vi "NeoShutdown.vi"(4 "Error In":errorcluster) -> (0 "ErrorOut":errorcluster)   [LabVIEW 2014]
panel:
  out "Close: status":i32
  out "Status: clear all buffers":i32
  in  "Handle":i32
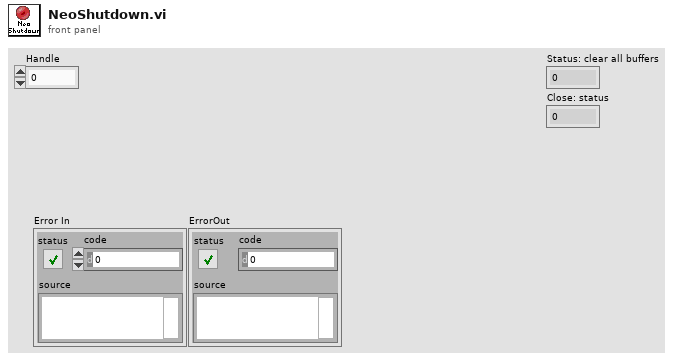
[diagram p1: front panel]
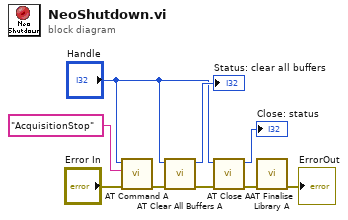
[diagram p0: block diagram]
diagram:
  n1 = call <userlib>:"AT Command A.vi"("error in (no error)"="Error In", "Feature"="AcquisitionStop" ("Command"), "Handle"="Handle") -> ("error out"=w2:errorcluster)  [unwired: 7 in, 1 out]
  n2 = call <userlib>:"AT Clear All Buffers A.vi"("error in (no error)"=w2, "Handle"="Handle") -> ("error out"=w8:errorcluster, "Status"=→"Status: clear all buffers":i32)  [unwired: 8 in]
  n3 = call <userlib>:"AT Close A.vi"("error in (no error)"=w8, "Handle"="Handle") -> ("error out"=w9:errorcluster, "Status"=→"Close: status":i32)  [unwired: 8 in]
  n4 = call <userlib>:"AT Finalise Library A.vi"("error in (no error)"=w9) -> ("error out"=→"ErrorOut":errorcluster)  [unwired: 9 in, 1 out]
